vi "system_UserConfigure.vi"() -> ()   [LabVIEW 2013, in "0_SystemCOnfiguration.lvlib"]
uses:
  0_Class/3_method/0_SystemConfiguration/system_Config.ctl
  2_Control/ProductType.ctl
  2_Control/PathControl.ctl
  0_SystemCOnfiguration.lvlib
panel:
  in  "Configuration":T1
  in  "OK Button":bool
  in  "Cancel Button":bool
  # "Function Configuration"
  # "Temprary Configuration"
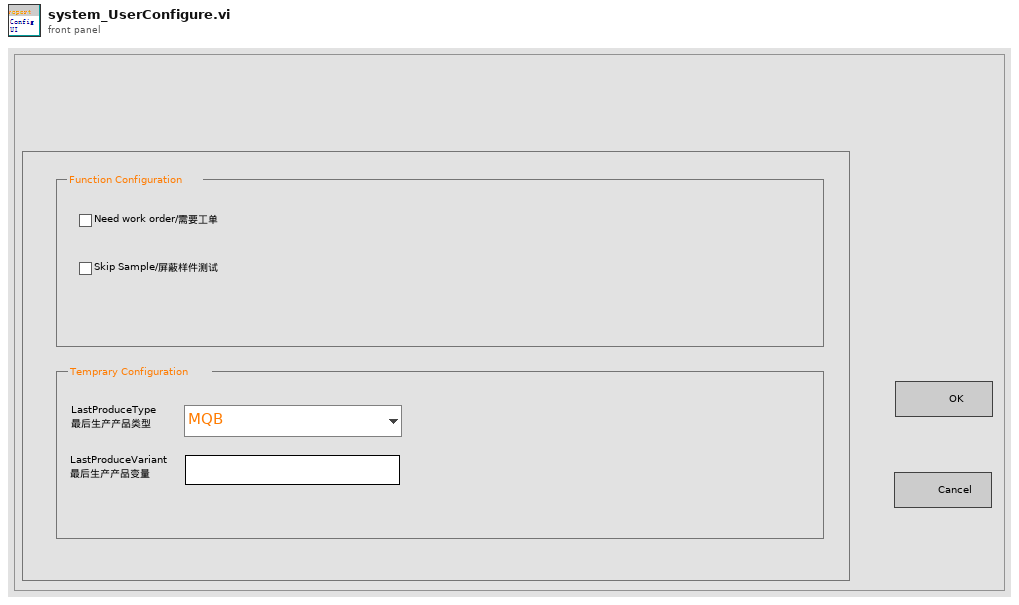
[diagram p1: front panel]
types:
  T1 = typedef "system_Config.ctl" = cluster{"Need work order":bool, "LastTestVariant":string, "Skip Sample":bool, "LastTestType":T2}
  T2 = typedef "ProductType.ctl" = enum16{"MQB", "Geely", "Volvo"}
  T3 = typedef "PathControl.ctl" = enum16{"UI_Banner_Path", "UI_Banner_Path1", "UI_Banner_Path2", "UI_Banner_Path0", "Menu_Manager_Run", "Menu_Debug", "Menu_Operater", "Path_ConfigFolder", "Path_Settings", "Path_Limits", "Path_TestItems", "Path_Company_logo", "Path_UUT", "Path_Customer_logo", "Path_Log_Folder", "Path_Log_Single_Folder", "Path_Config_DB", "Path_TestItem", "Path_TestLimit_Head", "Path_Log_Template", "Path_ExcelLog_Template", "Path_Label", "Path_Manual_Lable", "Path_Manual_TypeConfig", "Path_Message", "Path_ErrorLog_Folder"}
  T4 = enum16{"open", "replace", "create", "open or create", "replace or create", "replace or create with confirmation"}
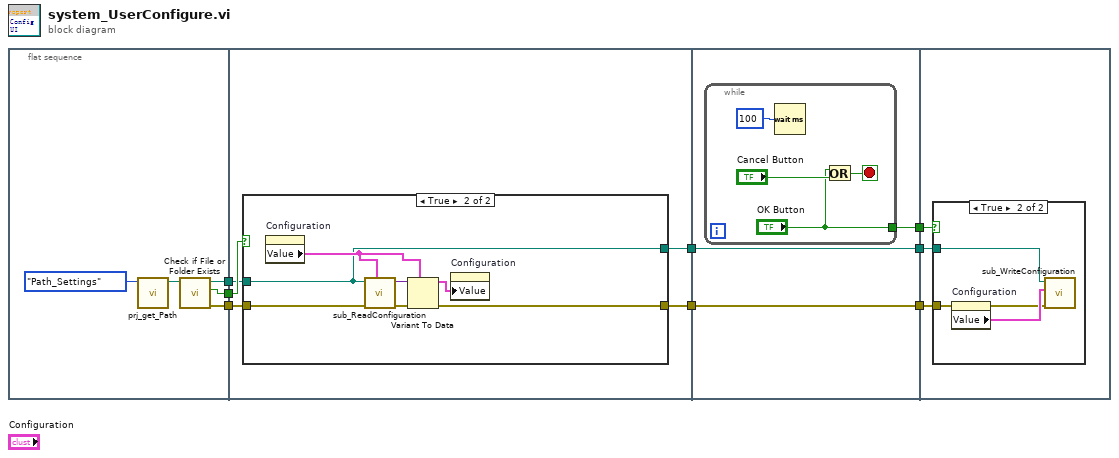
[diagram p0: block diagram]
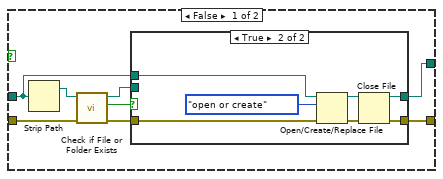
[diagram p2: hidden frame]
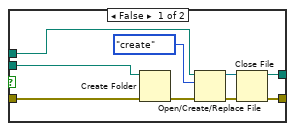
[diagram p3: hidden frame]
diagram:
  n1 = flat-sequence {
    tunnel: [w13] -> w8
    tunnel: [w12] -> w7
    tunnel: [w11] -> w6
    tunnel: w8 -> [w18]
    tunnel: w7 -> [w17]
    tunnel: w6 -> [w16]
    tunnel: [w15] -> w5
    tunnel: [w14] -> w2
    tunnel: [w52] -> w4
    tunnel: w5 -> [w51]
    tunnel: [w51] -> w3
    tunnel: w2 -> [w50]
    tunnel: [w50] -> w1
    tunnel: w3 -> [w58]
    tunnel: w4 -> [w59]
    tunnel: w1 -> [w57]
    frame #0 {
      n2 = call "prj_get_Path.vi"("Path_Item"=PathControl."Path_Settings") -> ("Detail path"=w10:path)  [unwired: 10 in]
      n3 = call <vilib>:"Check if File or Folder Exists.vi"("path"=w10) -> ("error out"=w11:errorcluster, "file or folder exists?"=w13:bool, "dup path"=w12:path)  [unwired: 8 in]
    }
    frame #1 {
      n4 = case shown="True" w18 {
        tunnel: w17 -> [w20 w44]
        tunnel: w16 -> [w25 w48]
        tunnel: [w19 w44] -> w15
        tunnel: [w21 w43] -> w14
        frame False {
          n5 = Strip Path(path=w20) -> (stripped path=w26:path)  [unwired: 1 out]
          n6 = call <vilib>:"Check if File or Folder Exists.vi"("error in (no error)"=w25, "path"=w26) -> ("error out"=w23:errorcluster, "file or folder exists?"=w24:bool, "dup path"=w22:path)  [unwired: 7 in]
          n7 = case shown="True" w24 {
            tunnel: w20 -> [w33 w42]
            tunnel: w23 -> [w34 w40]
            tunnel: w22 -> [w35 _]
            tunnel: [w28 w37] -> w21
            tunnel: [w27 w36] -> w19
            frame False {
              n8 = Create Folder(path (use dialog)=w35, error in=w34) -> (error out=w31:errorcluster)  [unwired: 1 in, 2 out]
              n9 = Open/Create/Replace File(file path (use dialog)=w33, error in=w31, operation (0:open)=T4."create" ("操作(0:open)")) -> (refnum out=w30:refnum<file>, error out=w29:errorcluster)  [unwired: 3 in, 1 out]
              n10 = Close File(refnum=w30, error in=w29) -> (path=w27:path, error out=w28:errorcluster)
            }
            frame True {
              n11 = Open/Create/Replace File(file path (use dialog)=w42, error in=w40, operation (0:open)=T4."open or create" ("操作(0:open)")) -> (refnum out=w39:refnum<file>, error out=w38:errorcluster)  [unwired: 3 in, 1 out]
              n12 = Close File(refnum=w39, error in=w38) -> (path=w36:path, error out=w37:errorcluster)
            }
          }
        }
        frame True {
          n13 = property on="Configuration" class="Clust (strict)"() -> ("Value"=w47:T1)  [unwired: 2 in, 2 out]
          n14 = call "sub_ReadConfiguration.vi"("Section Formatted Cluster Type"=w47, "error in (no error)"=w48, "configuration file path"=w44) -> ("error out"=w45:errorcluster, "数据"=w46:variant)  [unwired: 7 in]
          n15 = Variant To Data(error in=w45, type=w47, Variant=w46) -> (data=w49:T1, error out=w43:errorcluster)
          n16 = property on="Configuration" class="Clust (strict)"("Value"=w49) -> ()  [unwired: 2 in, 2 out]
        }
      }
    }
    frame #2 {
      n17 = while {
        tunnel: ["OK Button"] -> w52
        stop <- w55 stop-if-true
        n18 = Wait (ms)(milliseconds to wait=100) -> ()  [unwired: 1 out]
        n19 = Or(x="OK Button", y="Cancel Button") -> (x .or. y?=w55:bool)
      }
    }
    frame #3 {
      n20 = case shown="True" w59 {
        tunnel: w58 -> [_ w62]
        tunnel: w57 -> [_ w60]
        frame False {
        }
        frame True {
          n21 = property on="Configuration" class="Clust (strict)"(error in=w60) -> (error out=w61:errorcluster, "Value"=w63:T1)  [unwired: 1 in, 1 out]
          n22 = call "sub_WriteConfiguration.vi"("error in (no error)"=w61, "INI Fomatted Cluster"=w63, "configuration file path"=w62) -> ()  [unwired: 8 in, 1 out]
        }
      }
    }
  }
